vi "ni579x Configure Reference Level.vi"(0 "Register Bus":T5, 1 "scope":string="rx", 5 "reference level [dBm]":dbl, 7 "headroom [dB]":dbl, 9 "frequency [Hz]":dbl format="%#_6p", 11 "Error In":errorcluster, 12 "characterization data":T2 {"Frequencies [Hz]" format="%#_6p"}, 13 "correct IQ imbalance?":bool=TRUE) -> (4 "Register Bus (out)":T5, 6 "coerced reference level [dBm]":dbl, 8 "coerced vertical range [Vpp]":dbl format="%#_6p", 10 "IQ impairment correction":T1, 15 "Error Out":errorcluster)   [LabVIEW 2015, in "ni579x Config v2 Host.lvlib"]
doc: "Configures the Rx front end attenuators and filters to achieve the specified reference level, returns the IQ impairment correction data which can be used to correct IQ impairments, and returns the resulting vertical range that can be used to scale binary data retrieved from the device. Also sets the RF filter appropriately for the specified frequency.\n\n<B>Input Parameters</B>\n\n<B>Register Bus</B> The Register Bus object created by the ni579x Open VI and used as the session handle for the NI-579x Configuration Design Library.\n\n<B>scope</B> Specifies which channel to configure. Can be \"rx\".\n\n<B>reference level [dBm]</B> Specifies the maximum power (in dBm) of the signals expected at the input terminal of the device. The RF signal path of the device will be configured to maximize the dynamic range of the measurement relative to this power level.\n\n<B>frequency [Hz]</B> Specifies the frequency the LO is tuned to for the measurement.\n\n<B>headroom [dB]</B> Specifies the amount of headroom to leave in the range of the ADC if the signal input to the device is at the reference level power. Useful to avoid clipping/overrange errors and DSP overflows.\n\n<B>correct IQ imbalance?</B> Specifies whether this VI should calculate the IQ impairment correction values. Set to false if you are not using the IQ impairment correction DSP blocks in the FPGA.\n\n<B>characterization data</B> A set of data that describes the characteristics of this device that allows the VI to calculate the proper attenuation and IQ imbalance correction settings for the specified frequency. This data is stored in the EEPROM and can be retrieved using the ni579x Load Characterization Data (EEPROM) VI. For the 5791, the Rx data is index 0 in the array of characterization data returned by ni579x Load Characterization Data (EEPROM).vi\n\n<B>Output Parameters</B>\n\n<B>Register Bus (out)</B> The Register Bus object created by the ni579x Open VI and used as the session handle for the NI-579x Configuration Design Library.\n\n<B>coerced reference level [dBm]</B> The actual reference level the device was configured to. This is the maximum power level that can be input to the device without exceeding the vertical range of the ADCs.\n\n<B>coerced vertical range [Vpp]</B> The peak-to-peak vertical range, in Volts, of the device as currently configured. You can use this value to scale binary data retrieved from the device to Volts. This value assumes that the IQ impairment correction values returned by this VI are applied to the signal using the IQ Impairment Correction DSP block in the FPGA.\n\n<B>IQ impairment correction</B> The values to apply to the IQ Impairment Correction DSP block in the FPGA, in order to correct gain and phase imbalances in the mixer."
uses:
  <instrlib>/ni579x/Config/v2/Host/ni579x Config v2 Host.lvlib
  <instrlib>/_niInstr/Register Bus/v0/Host/Public/Register Bus Session.ctl
  <instrlib>/_niInstr/Register Bus/v0/Host/Private/Session Data.ctl
  <instrlib>/ni579x/Config/v2/Shared/Types/ni579x Characterization Data.ctl
  <instrlib>/ni579x/Config/v2/Shared/Types/ni579x IQ Imbalance.ctl
  <instrlib>/ni579x/Config/v2/Shared/Types/ni579x Gain to Attenuation Mapping.ctl
  <instrlib>/_niInstr/DSP/v1/Shared/Public/IQ Impairments.ctl
  <instrlib>/_niInstr/DSP/v1/Shared/niInstr DSP v1 Shared.lvlib
  <instrlib>/ni579x/Config/v2/Shared/ni579x Config v2 Shared.lvlib
  <instrlib>/_niInstr/Register Bus/v0/Host/niInstr Register Bus v0 Host.lvlib
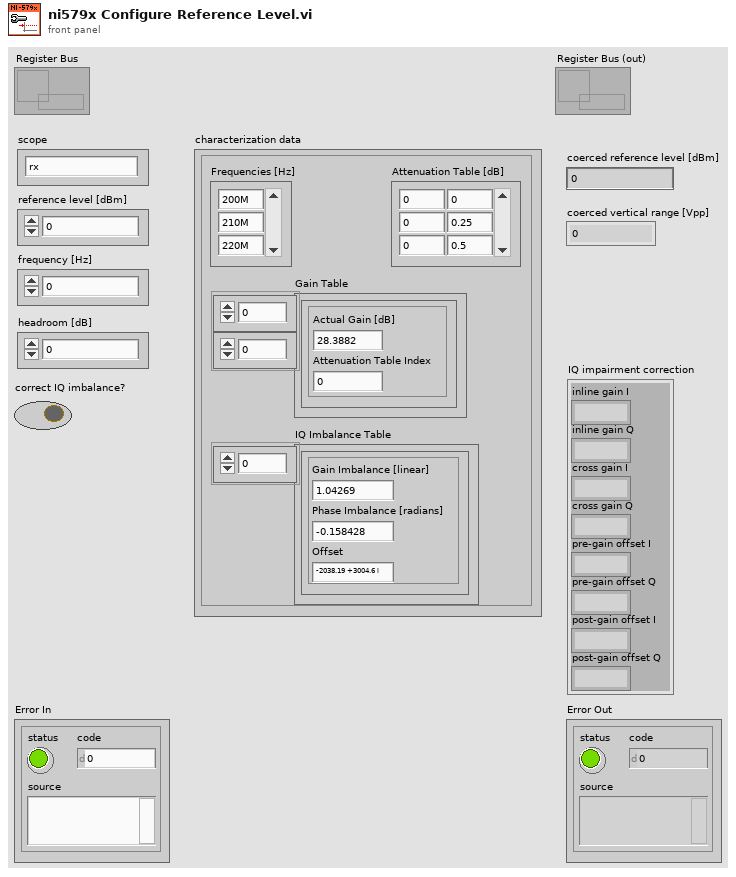
[diagram p1: front panel]
types:
  T1 = typedef "niInstr DSP v1 Shared.lvlib/IQ Impairments.ctl" = cluster{"inline gain I":fxp<+/-,18,1>, "inline gain Q":fxp<+/-,18,1>, "cross gain I":fxp<+/-,18,1>, "cross gain Q":fxp<+/-,18,1>, "pre-gain offset I":fxp<+/-,18,1>, "pre-gain offset Q":fxp<+/-,18,1>, "post-gain offset I":fxp<+/-,18,1>, "post-gain offset Q":fxp<+/-,18,1>}
  T2 = typedef "ni579x Config v2 Shared.lvlib/ni579x Characterization Data.ctl" = cluster{"Attenuation Table [dB]":dbl[][], "Frequencies [Hz]":dbl[], "IQ Imbalance Table":T3[], "Gain Table":T4[][]}
  T3 = typedef "ni579x Config v2 Shared.lvlib/ni579x IQ Imbalance.ctl" = cluster{"Gain Imbalance [linear]":dbl, "Phase Imbalance [radians]":dbl, "Offset":cdb}
  T4 = typedef "ni579x Config v2 Shared.lvlib/ni579x Gain to Attenuation Mapping.ctl" = cluster{"Actual Gain [dB]":dbl, "Attenuation Table Index":i32}
  T5 = typedef "niInstr Register Bus v0 Host.lvlib/Register Bus Session.ctl" = refnum<queue>
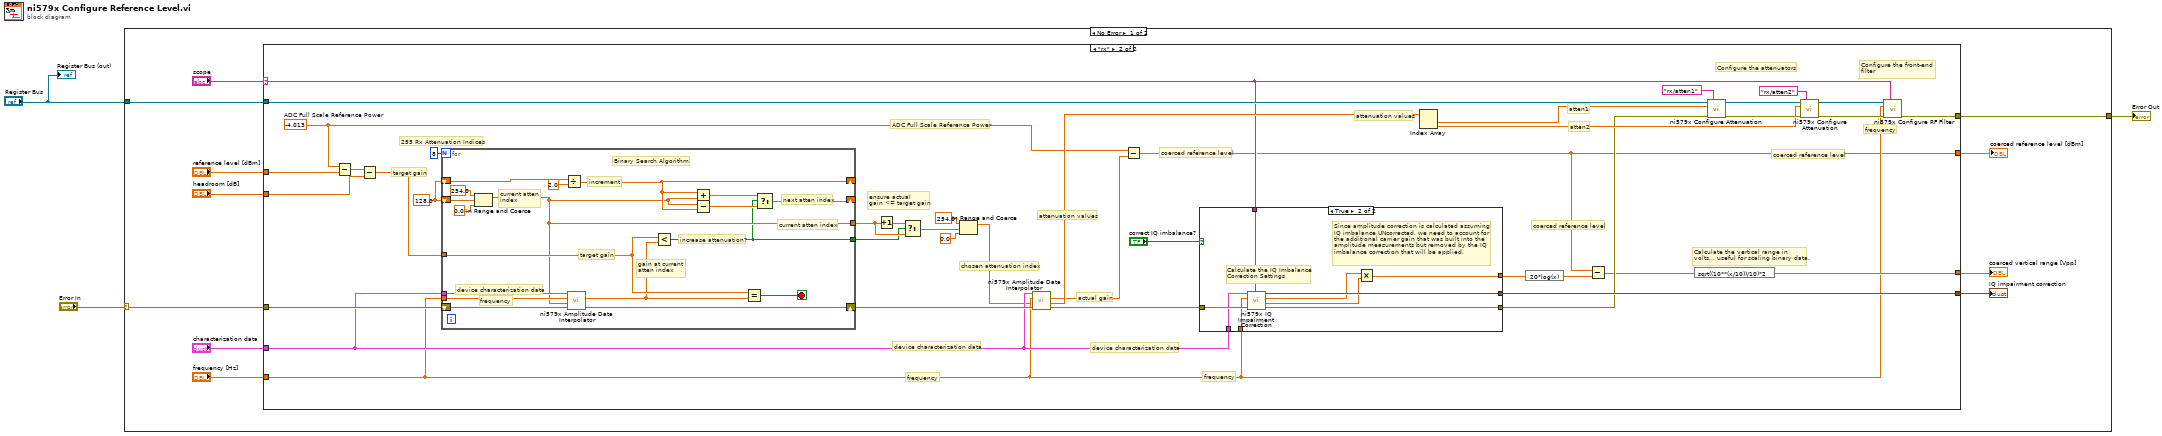
[diagram p0: block diagram]
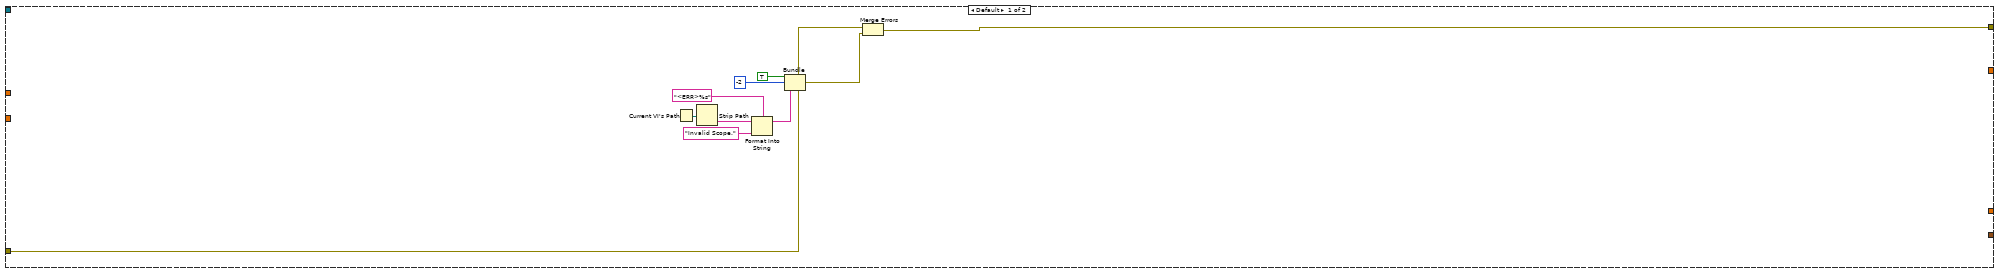
[diagram p2: hidden frame]
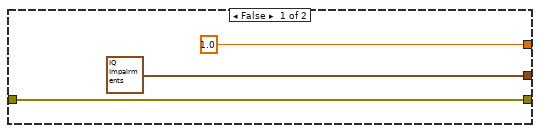
[diagram p3: hidden frame]
diagram:
  n1 = case shown="No Error" "Error In" {
    selector: "Error In" -> [w9 w95]
    tunnel: [w7 w95] -> w2
    tunnel: "Register Bus" -> [w10 _]
    frame No Error {
      n2 = case shown="\"rx\"" "scope" {
        selector: "scope" -> [_ w35]
        tunnel: "reference level [dBm]" -> [_ w63]
        tunnel: "frequency [Hz]" -> [_ w34]
        tunnel: "characterization data" -> [_ w41]
        tunnel: w10 -> [_ w64]
        tunnel: w9 -> [w16 w59]
        tunnel: [_ w26] -> w8
        tunnel: [w15 w37] -> w7
        tunnel: "headroom [dB]" -> [_ w61]
        tunnel: [_ w56] -> w5
        tunnel: [_ w40] -> w4
        frame Default {
          n3 = Current VI's Path() -> (path=w18:path)
          n4 = Strip Path(path=w18) -> (name=w19:string)  [unwired: 1 out]
          n5 = Format Into String(format string="<ERR>%s", initial string=w19, "Invalid Scope." ("input 1")) -> (resulting string=w20:string)  [unwired: 1 in, 1 out]
          n6 = Bundle(cluster=w16, "status"=TRUE, "code"=-2, "source"=w20) -> (w21:errorcluster)
          n7 = Merge Errors(w16, w21) -> (w15:errorcluster)
        }
        frame "rx" {
          w58 = 128.0
          w42 = -4.013  # ADC Full Scale Reference Power
          # "coerced reference level"
          # "coerced reference level"
          # "coerced reference level"
          # "attenuation values"
          # "frequency"
          # "Configure the front-end\nfilter"
          # "Calculate the vertical range in \nvolts... useful for scaling binary data."
          # "device characterization data"
          # "frequency"
          # "device characterization data"
          # "frequency"
          # "Configure the attenuators"
          # "atten2"
          # "atten1"
          # "ADC Full Scale Reference Power"
          # "attenuation values"
          # "actual gain"
          # "chosen attenuation index"
          # "ensure actual \ngain <= target gain"
          # "target gain"
          # "255 Rx Attenuation Indices"
          n8 = Subtract(x=w42, y=w63) -> (x-y=w62:dbl)
          n9 = Subtract(x=w62, y=w61) -> (x-y=w60:dbl)
          n10 = for {
            N: 8 ("255 of RX Attenuation Indices") -> [_]
            tunnel: w41 -> [w84]
            tunnel: w34 -> [w83]
            tunnel: w60 -> [w85]
            shift-right: [w93] -> w46
            shift-left: w59 -> [w94]
            shift-right: [w87] -> _
            shift-left: w58 -> [w79]
            shift-right: [w86] -> _
            shift-left: w58 -> [w89]
            tunnel: [w78] -> w47
            tunnel: [w77] -> w39
            stop <- w92 stop-if-true
            # "device characterization data"
            # "frequency"
            # "target gain"
            # "gain at current \natten index"
            # "current atten index"
            # "next atten index"
            # "increase attenuation?"
            # "increment"
            # "current atten\nindex"
            # "Binary Search Algorithm"
            n11 = In Range and Coerce(upper limit=254.0, x=w79, lower limit=0.0) -> (coerced(x)=w78:dbl)  [unwired: 1 out]
            n12 = Divide(x=w89, y=2.0) -> (x/y=w86:dbl)
            n13 = call <instrlib>:"ni579x Amplitude Data Interpolator.vi"("Error In"=w94, "attenuation index"=w78, "frequency [Hz]"=w83, "characterization data"=w84) -> ("Error Out"=w93:errorcluster, "amplitude data"=w82:dbl)  [unwired: 5 in, 1 out]
            n14 = Less?(x=w85, y=w82) -> (x < y?=w77:bool)
            n15 = Add(x=w86, y=w78) -> (x+y=w91:dbl)
            n16 = Subtract(x=w78, y=w86) -> (x-y=w90:dbl)
            n17 = Equal?(x=w85, y=w82) -> (x = y?=w92:bool)
            n18 = Select(t=w91, s=w77, f=w90) -> (s? t:f=w87:dbl)
          }
          n19 = Increment(x=w47) -> (x+1=w57:dbl)
          n20 = Select(t=w57, s=w39, f=w47) -> (s? t:f=w31:dbl)
          n21 = In Range and Coerce(upper limit=254.0, x=w31, lower limit=0.0) -> (coerced(x)=w30:dbl)  [unwired: 1 out]
          n22 = call <instrlib>:"ni579x Amplitude Data Interpolator.vi"("Error In"=w46, "attenuation index"=w30, "frequency [Hz]"=w34, "characterization data"=w41) -> ("Error Out"=w45:errorcluster, "attenuator values [dB]"=w44:dbl[], "amplitude data"=w43:dbl)  [unwired: 5 in]
          n23 = Subtract(x=w42, y=w43) -> (x-y=w26:dbl)
          n24 = case shown="True" "correct IQ imbalance?" {
            tunnel: [T1 {"inline gain I"=0.9999923706054688, "inline gain Q"=0.9999923706054688, "cross gain I"=0.0, "cross gain Q"=0.0, "pre-gain offset I"=0.0, "pre-gain offset Q"=0.0, "post-gain offset I"=0.0, "post-gain offset Q"=0.0} ("IQ impairment") w76] -> w56
            tunnel: [w67 w75] -> w49
            tunnel: w45 -> [w67 w74]
            tunnel: w41 -> [_ w73]
            tunnel: w35 -> [_ w72]
            tunnel: w34 -> [_ w71]
            tunnel: [1.0 ("correction gain") w68] -> w25
            frame False {
            }
            frame True {
              # "Since amplitude correction is calculated assuming\nIQ imbalance UNcorrected, we need to account for\nthe additional carrier gain that was built into the\namplitude measurements but removed by the IQ\nimbalance correction that will be applied."
              # "Calculate the IQ Imbalance\nCorrection Settings"
              n25 = call <instrlib>:"ni579x IQ Impairment Correction.vi"("scope"=w72, "Error In"=w74, "frequency [Hz]"=w71, "characterization data"=w73) -> ("Error Out"=w75:errorcluster, "uncorrected carrier gain"=w69:dbl, "correction gain"=w70:dbl, "IQ impairment correction out"=w76:T1)  [unwired: 4 in]
              n26 = Multiply(x=w70, y=w69) -> (x*y=w68:dbl)
            }
          }
          n27 = Index Array(array=w44) -> (element #1=w51:dbl, element #2=w50:dbl)  [unwired: 2 in]
          n28 = expression code="20*log(x)"(w25) -> (w28:dbl)
          n29 = Subtract(x=w26, y=w28) -> (x-y=w29:dbl)
          n30 = expression code="sqrt((10**(x/10))/10)*2"(w29) -> (w40:dbl)
          n31 = call <instrlib>:"ni579x Configure Attenuation.vi"("Register Bus"=w64, "scope"="rx/atten1", "attenuation [dB]"=w51, "Error In"=w49) -> ("Register Bus (out)"=w53:T5, "Error Out"=w52:errorcluster)  [unwired: 9 in, 1 out]
          n32 = call <instrlib>:"ni579x Configure Attenuation.vi"("Register Bus"=w53, "scope"="rx/atten2", "attenuation [dB]"=w50, "Error In"=w52) -> ("Register Bus (out)"=w36:T5, "Error Out"=w38:errorcluster)  [unwired: 9 in, 1 out]
          n33 = call <instrlib>:"ni579x Configure RF Filter.vi"("Register Bus"=w36, "scope"=w35, "frequency [Hz]"=w34, "Error In"=w38) -> ("Error Out"=w37:errorcluster)  [unwired: 9 in, 2 out]
        }
      }
      "IQ impairment correction" <- w5
      "coerced reference level [dBm]" <- w8
      "coerced vertical range [Vpp]" <- w4
    }
    frame Error {
    }
  }
  "Error Out" <- w2
  "Register Bus (out)" <- "Register Bus"
